vi "testionsource.vi"() -> ()   [LabVIEW 2014, in "Panels.lvlib"]
uses:
  Panels.lvlib
  CSlibraries-extern/DimLVEvent/DimIndicators/DimIndicators.lvlib
  CS_Core/CSSystem/CoreLib/CoreLib.lvlib
  CSlibraries/UtilityLib/UtilityLib.valueStatus.ctl
  CSlibraries/UtilityLib/UtilityLib.lvlib
  CSlibraries-extern/DimLVEvent/LVDimInterface/LVDimInterface.lvlib
  Instance           1 21Saved   testionsource .vi
  CSlibraries-extern/DimLVEvent/DimIndicators/DimIndicators.numericType.ctl
  CSlibraries-extern/DimLVEvent/DimIndicators/DimIndicators.numericArrayType.ctl
  CSlibraries-extern/DimLVEvent/DimIndicators/DimIndicators.anyType.ctl
panel:
  in  "SetFileLocation_Data":T1={"data"="NOLINK", "no link"=TRUE, "quality"=-1, "timeStamp"=0.0}
  in  "ISMFfreq":bool
  out "ISMFfreq_Mon":dbl=inf format="%.4f"
  in  "ISMFOffset":bool
  out "ISMFOffset_Mon":dbl=inf format="%.4f"
  in  "ISMFfreq_MonData":T2={"data"=inf, "no link"=FALSE, "quality"=1, "timeStamp"=3269018078.71}
  in  "ISMFalpha_SetValueInfoData":T3={"data"=[-1000.0, 1000.0, -1.0], "no link"=FALSE, "quality"=0, "timeStamp"=3269018078.694}
  in  "ISMFalpha_SetData":T3={"data"=[0.0, 0.0, 0.0, 0.0], "no link"=FALSE, "quality"=1, "timeStamp"=3269018077.397}
  in  "ISMFalpha_MonData":T2={"data"=inf, "no link"=TRUE, "quality"=-1, "timeStamp"=0.0}
  in  "ISMFalpha":bool
  out "ISMFalpha_Mon":dbl=inf format="%.4f"
  in  "SetFileLocation":path=path "\\\\intranet\\Files/projects/lebit/Data Exchange/data/TSTControl"
  in  "TSTBase_SetValueInfoData":T3={"data"=[-1000.0, 1000.0, -1.0], "no link"=FALSE, "quality"=0, "timeStamp"=3269018078.694}
  in  "ISMFDC":bool
  in  "ISMFamp":bool
  in  "ISMFDC_SetValueInfoData":T3={"data"=[0.0, 10.0, -1.0], "no link"=FALSE, "quality"=0, "timeStamp"=3269018078.71}
  out "i ref out":refnum<vi>
  in  "Last Loaded File_Data":T1={"data"="NOLINK", "no link"=TRUE, "quality"=-1, "timeStamp"=0.0}
  out "FileUpToDate":bool=TRUE caption="Parameter Changed"
  in  "Close All Panels":bool
  in  "ISMFfreq_SetValueInfoData":T3={"data"=[0.0, 10.0, -1.0], "no link"=FALSE, "quality"=0, "timeStamp"=3269018078.694}
  in  "ISMFOffset_SetValueInfoData":T3={"data"=[-10.0, 10.0, -1.0], "no link"=FALSE, "quality"=0, "timeStamp"=3269018078.71}
  in  "ISMFamp_SetValueInfoData":T3={"data"=[0.0, 10.0, -1.0], "no link"=FALSE, "quality"=0, "timeStamp"=3269018078.694}
  in  "ISMFamp_SetData":T3={"data"=[0.0, 0.0, 0.0, 0.0], "no link"=FALSE, "quality"=1, "timeStamp"=3269018077.507}
  in  "ISMFOffset_SetData":T3={"data"=[0.0, 0.0, 0.0, 0.0], "no link"=FALSE, "quality"=1, "timeStamp"=3269018077.507}
  in  "ISMFfreq_SetData":T3={"data"=[0.0, 0.0, 0.0, 0.0], "no link"=FALSE, "quality"=1, "timeStamp"=3269018077.507}
  in  "ISMFDC_SetData":T3={"data"=[0.0, 0.0, 0.0, 0.0], "no link"=FALSE, "quality"=1, "timeStamp"=3269018077.507}
  out "Last Loaded File":string
  in  "ISMFDC_MonData":T2={"data"=inf, "no link"=FALSE, "quality"=1, "timeStamp"=3269018078.71}
  in  "ISMFamp_MonData":T2={"data"=inf, "no link"=FALSE, "quality"=1, "timeStamp"=3269018078.694}
  in  "ISMFOffset_MonData":T2={"data"=inf, "no link"=FALSE, "quality"=1, "timeStamp"=3269018078.71}
  out "ISMFDC_Mon":dbl=inf format="%.4f"
  out "ISMFamp_Mon":dbl=inf format="%.4f"
  # "Parameter changed, data file is no longer up-to-date."
  # "Values in italic don't have a real monitor"
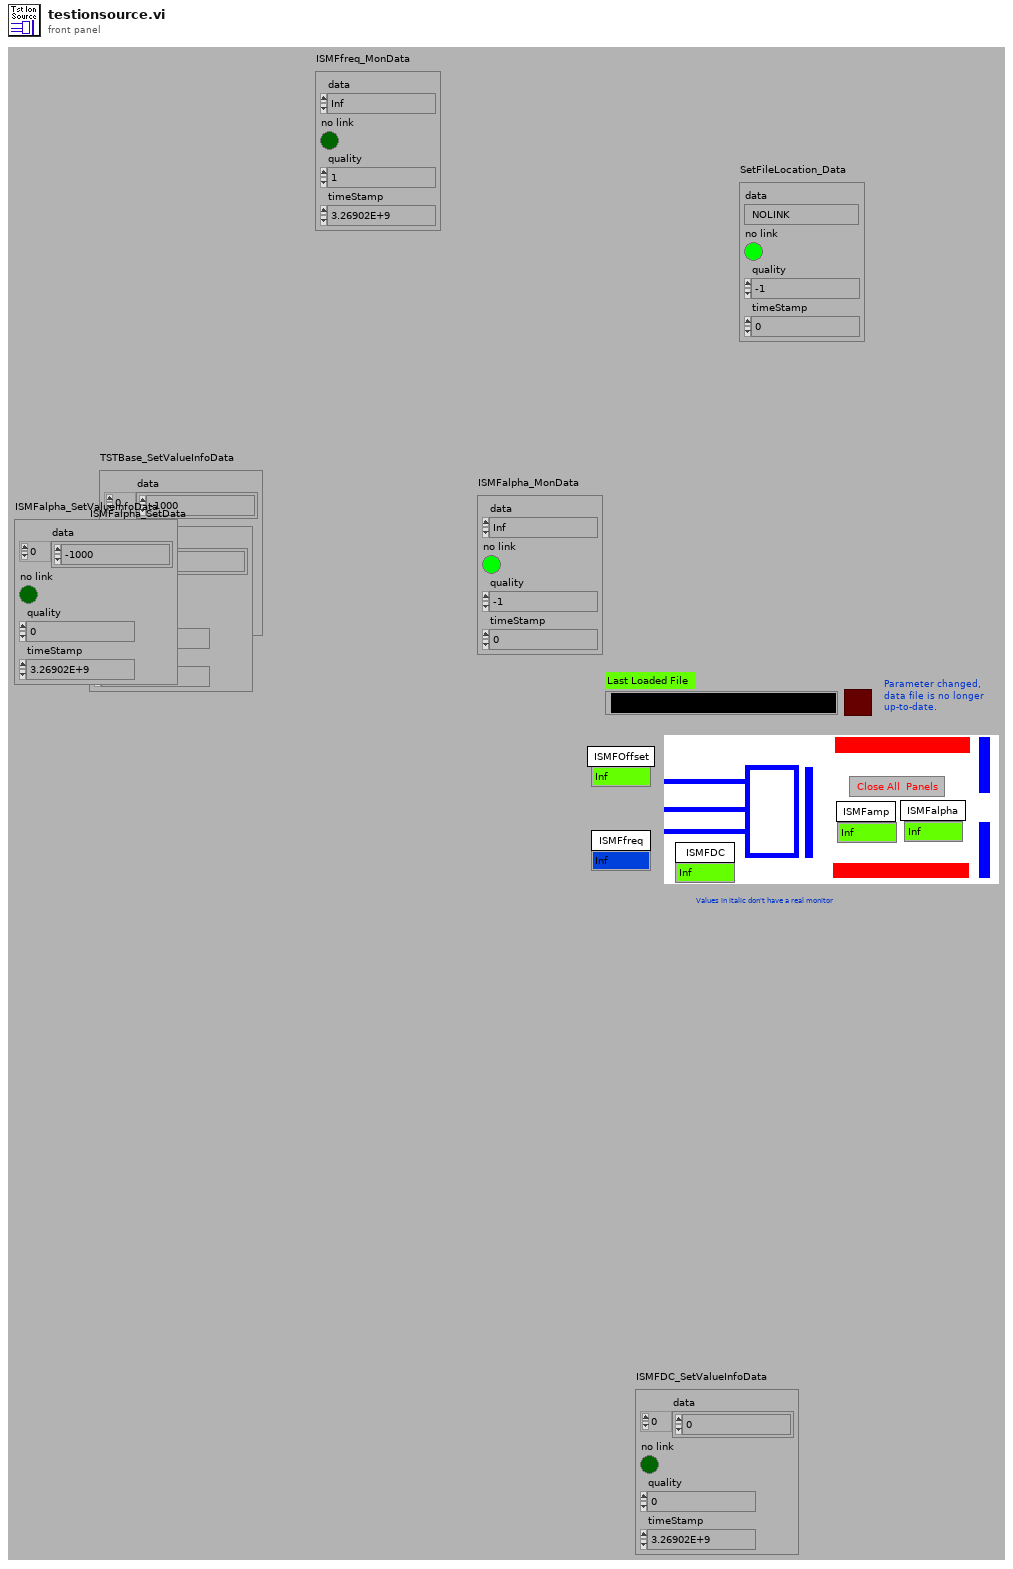
[diagram p1: front panel]
types:
  T1 = typedef "DimIndicators.lvlib/DimIndicators.anyType.ctl" = cluster{"data":string, "no link":bool, "quality":i32, "timeStamp":dbl}
  T2 = typedef "DimIndicators.lvlib/DimIndicators.numericType.ctl" = cluster{"data":dbl, "no link":bool, "quality":i32, "timeStamp":dbl}
  T3 = typedef "DimIndicators.lvlib/DimIndicators.numericArrayType.ctl" = cluster{"data":dbl[], "no link":bool, "quality":i32, "timeStamp":dbl}
  T4 = typedef "UtilityLib.lvlib/UtilityLib.valueStatus.ctl" = enum16{"no info available", "stand by/off", "on", "warning", "alarm/malfunction", "not implemented", "user action required", "important information", "system default", "control default", "indicator default", "button default"}
  T5 = cluster{"data":string, "no link":bool, "quality":i32, "timeStamp":dbl}
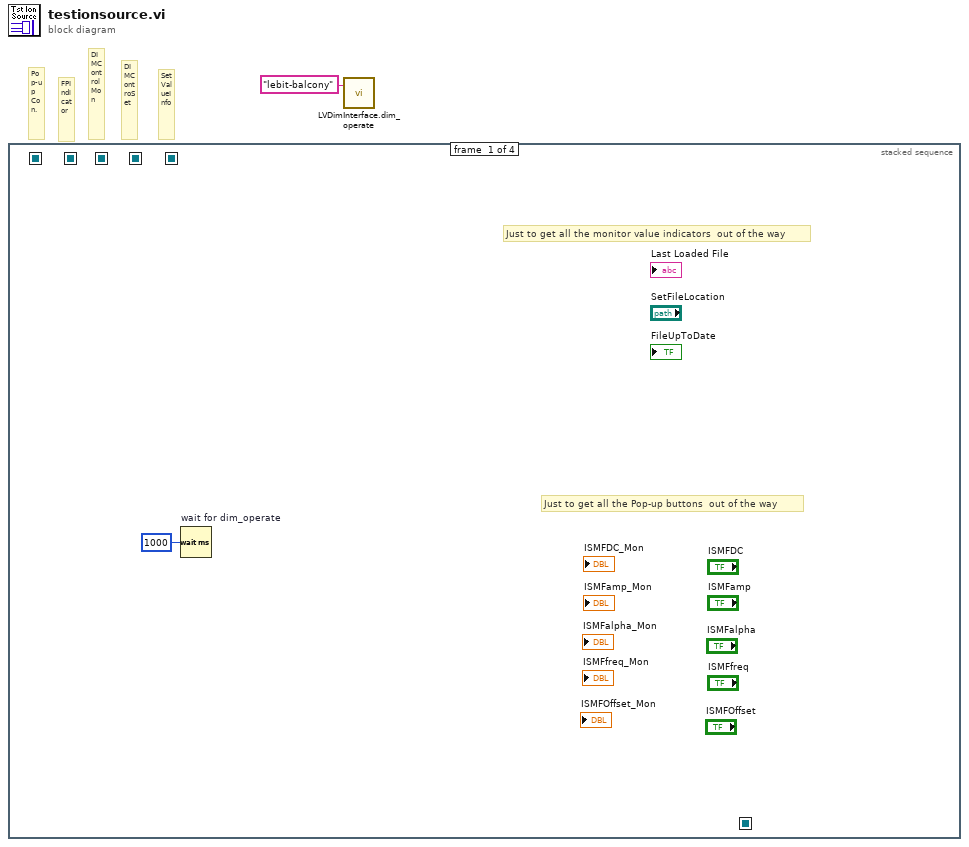
[diagram p0: block diagram]
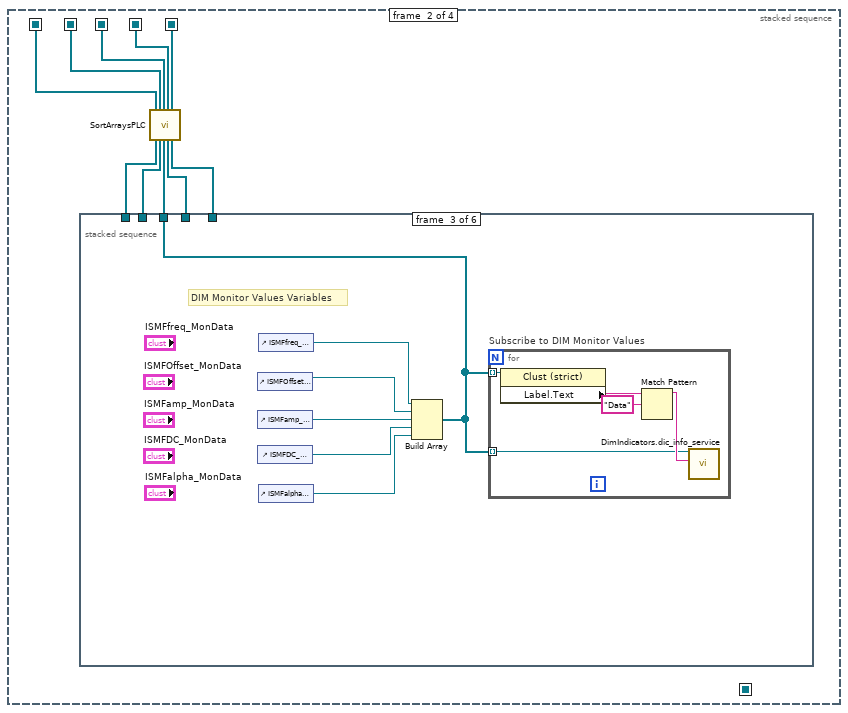
[diagram p2: hidden frame]
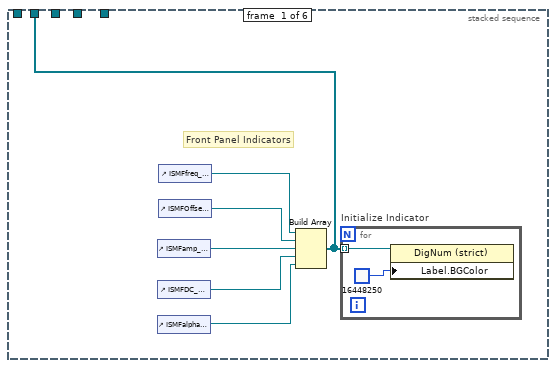
[diagram p3: hidden frame]
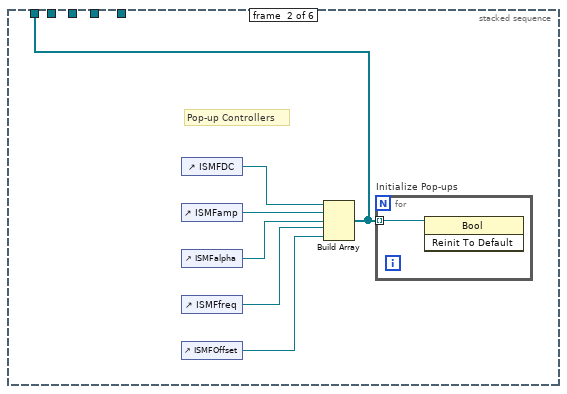
[diagram p4: hidden frame]
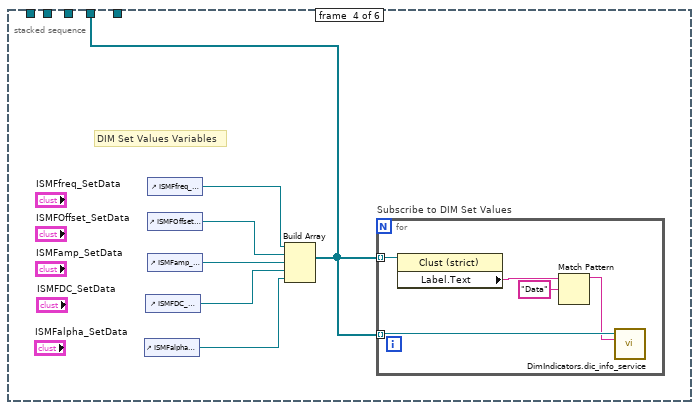
[diagram p5: hidden frame]
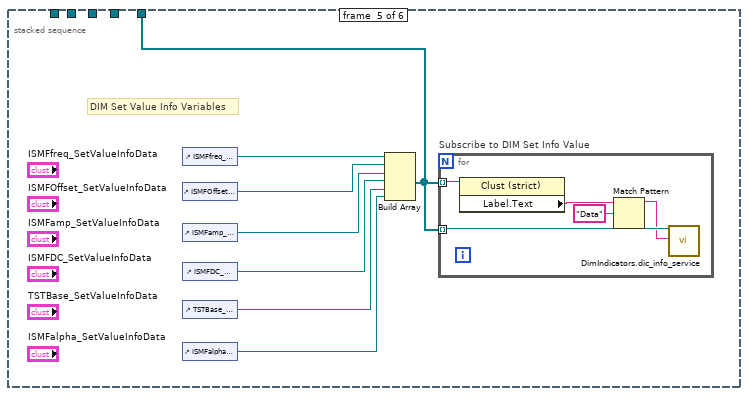
[diagram p6: hidden frame]
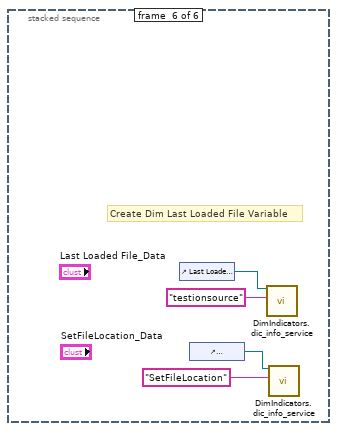
[diagram p7: hidden frame]
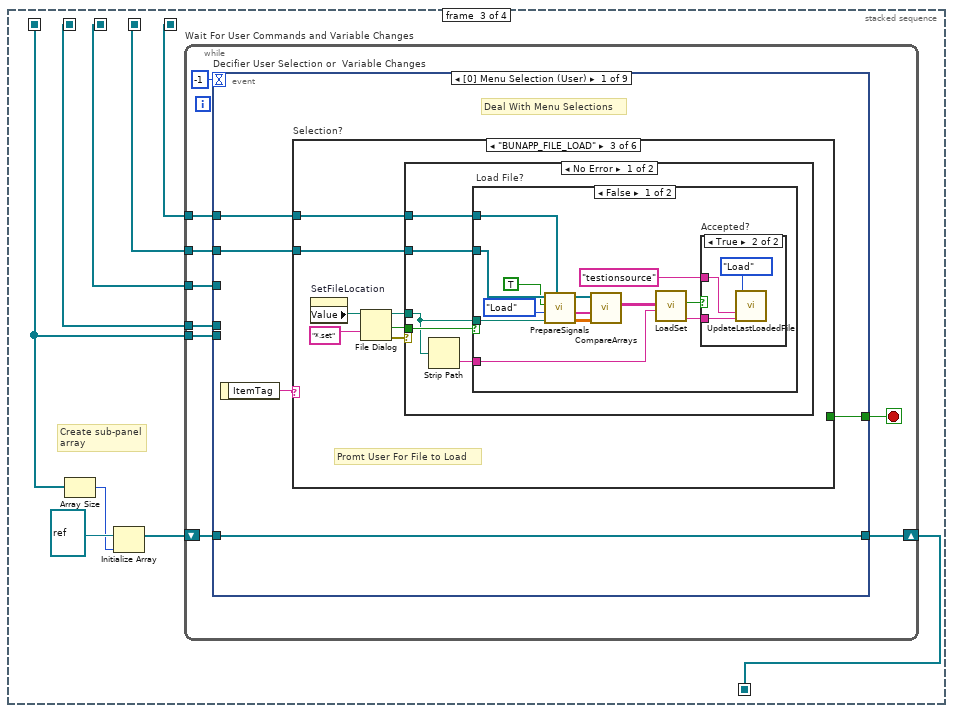
[diagram p8: hidden frame]
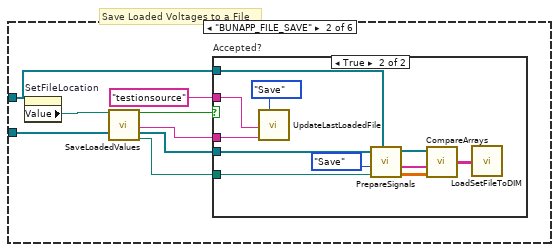
[diagram p10: hidden frame]
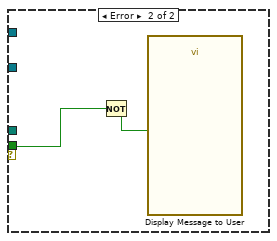
[diagram p14: hidden frame]
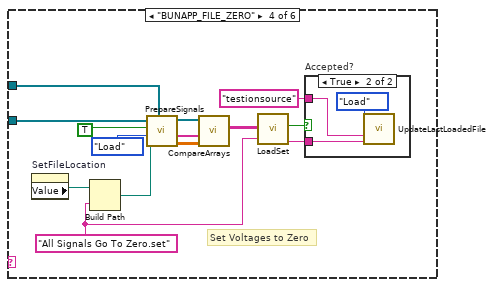
[diagram p15: hidden frame]
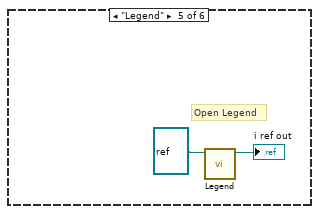
[diagram p17: hidden frame]
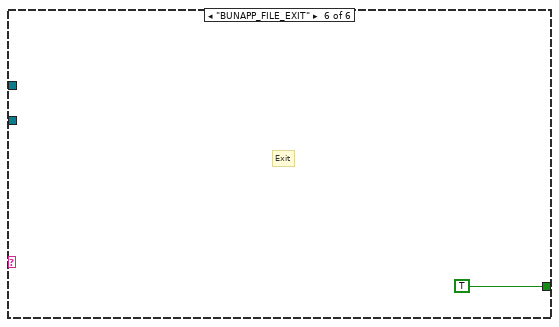
[diagram p18: hidden frame]
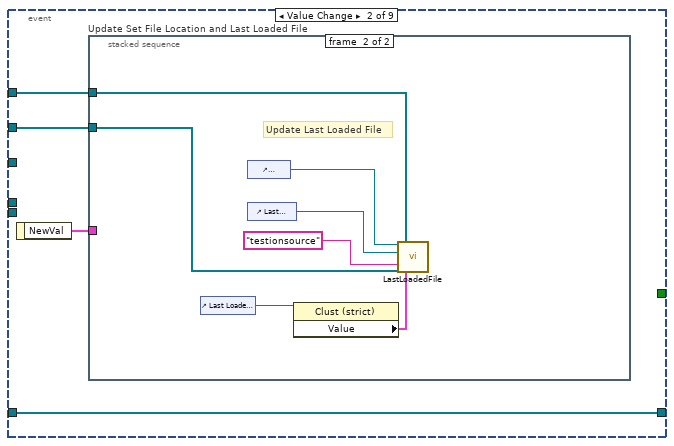
[diagram p19: hidden frame]
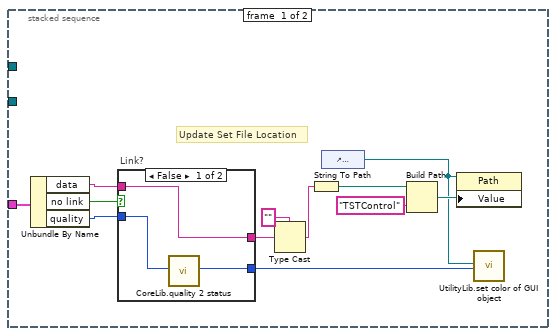
[diagram p20: hidden frame]
diagram:
  # "Pop-up Con."
  # "SetValueInfo"
  # "DIMControSet"
  # "DIMControlMon"
  # "FPIndicator"
  n1 = stacked-sequence {
    seq-local: [_ w6 _ _] -> [_ _ w71 _]
    seq-local: [_ w5 _ _] -> [_ _ w74 w268]
    seq-local: [_ _ w69 _] -> [_ _ _ w271]
    seq-local: [_ w4 _ _] -> [_ _ w68 w269]
    seq-local: [_ w3 _ _] -> [_ _ w67 w270]
    seq-local: [_ w7 _ _] -> [_ _ w66 _]
    frame #0 {
      # "Just to get all the Pop-up buttons  out of the way"
      # "Just to get all the monitor value indicators  out of the way"
      n2 = Wait (ms) "wait for dim_operate"(milliseconds to wait=u32 1000) -> ()  [unwired: 1 out]
    }
    frame #1 {
      # "Arrange references to all monitor-value related buttons into an array."
      n3 = stacked-sequence {
        tunnel: [w13 _ _ _ _ _] -> w11
        tunnel: [_ w21 _ _ _ _] -> w12
        tunnel: [_ _ w28 _ _ _] -> w10
        tunnel: [_ _ _ w39 _ _] -> w9
        tunnel: [_ _ _ _ w50 _] -> w8
        frame #0 {
          # "Front Panel Indicators"
          n4 = control-ref of="ISMFamp_Mon"() -> (w16:refnum<vi>)
          n5 = control-ref of="ISMFDC_Mon"() -> (w18:refnum<vi>)
          n6 = control-ref of="ISMFalpha_Mon"() -> (w17:refnum<vi>)
          n7 = control-ref of="ISMFfreq_Mon"() -> (w14:refnum<vi>)
          n8 = control-ref of="ISMFOffset_Mon"() -> (w15:refnum<vi>)
          n9 = Build Array(w14, w15, w16, w18, w17) -> (w13:refnum<vi>[])
          n10 = for "Initialize Indicator" {
            tunnel: w13 -> [w20] mode=indexing
            n11 = property on="Property Node" class="DigNum (strict)"(reference=w20, "Label.BGColor"=u32 16448250 ("Color Box")) -> ()  [unwired: 1 in, 2 out]
          }
        }
        frame #1 {
          # "Pop-up Controllers"
          n12 = control-ref of="ISMFDC"() -> (w26:refnum<vi>)
          n13 = control-ref of="ISMFamp"() -> (w25:refnum<vi>)
          n14 = control-ref of="ISMFalpha"() -> (w24:refnum<vi>)
          n15 = control-ref of="ISMFfreq"() -> (w23:refnum<vi>)
          n16 = control-ref of="ISMFOffset"() -> (w22:refnum<vi>)
          n17 = Build Array(w26, w25, w24, w23, w22) -> (w21:refnum<vi>[])
          n18 = for "Initialize Pop-ups" {
            tunnel: w21 -> [w27] mode=indexing
            n19 = invoke class="Bool" method="Reinit To Default"(reference=w27) -> ()  [unwired: 2 in, 3 out]
          }
        }
        frame #2 {
          # "DIM Monitor Values Variables"
          n20 = control-ref of="ISMFOffset_MonData"() -> (w33:refnum<vi>)
          n21 = control-ref of="ISMFamp_MonData"() -> (w32:refnum<vi>)
          n22 = control-ref of="ISMFDC_MonData"() -> (w31:refnum<vi>)
          n23 = control-ref of="ISMFfreq_MonData"() -> (w29:refnum<vi>)
          n24 = control-ref of="ISMFalpha_MonData"() -> (w30:refnum<vi>)
          n25 = Build Array(w29, w33, w32, w31, w30) -> (w28:refnum<vi>[])
          n26 = for "Subscribe to DIM Monitor Values" {
            tunnel: w28 -> [w35] mode=indexing
            tunnel: w28 -> [w34] mode=indexing
            n27 = property class="Clust (strict)"(reference=w34) -> ("Label.Text"=w37:string)  [unwired: 1 in, 2 out]
            n28 = Match Pattern(string=w37, regular expression="Data") -> (before substring=w36:string)  [unwired: 1 in, 3 out]
            n29 = call "DimIndicators.dic_info_service.vi"("controlRef"=w35, "serviceName"=w36) -> ()  [unwired: 16 in, 2 out]
          }
        }
        frame #3 {
          # "DIM Set Values Variables"
          n30 = control-ref of="ISMFalpha_SetData"() -> (w40:refnum<vi>)
          n31 = control-ref of="ISMFDC_SetData"() -> (w41:refnum<vi>)
          n32 = control-ref of="ISMFfreq_SetData"() -> (w44:refnum<vi>)
          n33 = control-ref of="ISMFOffset_SetData"() -> (w43:refnum<vi>)
          n34 = control-ref of="ISMFamp_SetData"() -> (w42:refnum<vi>)
          n35 = Build Array(w44, w43, w42, w41, w40) -> (w39:refnum<vi>[])
          n36 = for "Subscribe to DIM Set Values" {
            tunnel: w39 -> [w45] mode=indexing
            tunnel: w39 -> [w49] mode=indexing
            n37 = property class="Clust (strict)"(reference=w45) -> ("Label.Text"=w48:string)  [unwired: 1 in, 2 out]
            n38 = Match Pattern(string=w48, regular expression="Data") -> (before substring=w46:string)  [unwired: 1 in, 3 out]
            n39 = call "DimIndicators.dic_info_service.vi"("controlRef"=w49, "serviceName"=w46) -> ()  [unwired: 16 in, 2 out]
          }
        }
        frame #4 {
          # "DIM Set Value Info Variables"
          n40 = control-ref of="ISMFfreq_SetValueInfoData"() -> (w56:refnum<vi>)
          n41 = control-ref of="ISMFOffset_SetValueInfoData"() -> (w55:refnum<vi>)
          n42 = control-ref of="ISMFamp_SetValueInfoData"() -> (w54:refnum<vi>)
          n43 = control-ref of="ISMFDC_SetValueInfoData"() -> (w53:refnum<vi>)
          n44 = control-ref of="TSTBase_SetValueInfoData"() -> (w52:refnum<vi>)
          n45 = control-ref of="ISMFalpha_SetValueInfoData"() -> (w51:refnum<vi>)
          n46 = Build Array(w56, w55, w54, w53, w52, w51) -> (w50:refnum<vi>[])
          n47 = for "Subscribe to DIM Set Info Value" {
            tunnel: w50 -> [w57] mode=indexing
            tunnel: w50 -> [w61] mode=indexing
            n48 = property class="Clust (strict)"(reference=w57) -> ("Label.Text"=w60:string)  [unwired: 1 in, 2 out]
            n49 = Match Pattern(string=w60, regular expression="Data") -> (before substring=w58:string)  [unwired: 1 in, 3 out]
            n50 = call "DimIndicators.dic_info_service.vi"("controlRef"=w61, "serviceName"=w58) -> ()  [unwired: 16 in, 2 out]
          }
        }
        frame #5 {
          # "Create Dim Last Loaded File Variable"
          n51 = control-ref of="Last Loaded File_Data"() -> (w64:refnum<vi>)
          n52 = control-ref of="SetFileLocation_Data"() -> (w62:refnum<vi>)
          n53 = call "DimIndicators.dic_info_service.vi"("controlRef"=w64, "serviceName"="testionsource" ("string")) -> ()  [unwired: 16 in, 2 out]
          n54 = call "DimIndicators.dic_info_service.vi"("controlRef"=w62, "serviceName"="SetFileLocation" ("string")) -> ()  [unwired: 16 in, 2 out]
        }
      }
      n55 = call "SortArraysPLC.vi"("Pop-up Con."=w12, "FPIndicator in"=w11, "DIMControlMon"=w10, "DIMControSet"=w9, "SetValueInfo"=w8) -> ("Pop-up Con. out"=w7:refnum<vi>[], "FPIndicator out"=w6:refnum<vi>[], "DIMControlMon out"=w5:refnum<vi>[], "DIMControSet out"=w4:refnum<vi>[], "SetValueInfo out"=w3:refnum<vi>[])  [unwired: 18 in]
    }
    frame #2 {
      # "Create sub-panel\narray"
      n56 = Array Size(array=w66) -> (size(s)=w70:i32)
      n57 = Initialize Array(refnum<vi> refnum ("vi reference"), w70) -> (w73:refnum<vi>[])
      n58 = while "Wait For User Commands and Variable Changes" {
        tunnel: w74 -> [w82]
        tunnel: w71 -> [w81]
        shift-right: [w79] -> w69
        shift-left: w73 -> [w80]
        tunnel: w68 -> [w78]
        tunnel: w67 -> [w77]
        tunnel: w66 -> [w75]
        stop <- w83 stop-if-true
        n59 = event "Decifier User Selection or  Variable Changes" shown="[0] Menu Selection (User)" {
          selector: _ -> [_ _ _ _ _ _ _ _ _]
          dyn-events: _ -> [_ _ _ _ _ _ _ _ _]
          timeout: -1 -> [_ _ _ _ _ _ _ _ _]
          tunnel: [w85 _ _ _ _ _ _ _ _] -> w83
          tunnel: w82 -> [_ _ _ _ _ _ _ _ w245]
          tunnel: w81 -> [_ _ _ w195 _ _ _ _ _]
          tunnel: w80 -> [w88 w161 w192 w194 w222 w230 w237 w243 w244]
          tunnel: [w88 w161 w192 w194 w222 w228 w235 w243 _] -> w79
          tunnel: w78 -> [w86 w159 w190 _ w220 _ _ _ w246]
          tunnel: w77 -> [w84 w158 w186 _ _ _ _ _ w247]
          tunnel: w75 -> [_ _ _ _ _ w224 _ _ _]
          event Menu Selection (User) {
            # "Deal With Menu Selections"
            n60 = event-data() -> ("ItemTag"=w87:string)  [unwired: 1 in]
            n61 = case "Selection?" shown="\"BUNAPP_FILE_LOAD\"" w87 {
              tunnel: w86 -> [_ w93 w113 w151 _ _]
              tunnel: [_ _ _ _ _ TRUE ("stop")] -> w85
              tunnel: w84 -> [_ w89 w108 w138 _ _]
              frame "False", Default {
              }
              frame "BUNAPP_FILE_SAVE" {
                # "Save Loaded Voltages to a File"
                n62 = property on="SetFileLocation" class="Path"() -> ("Value"=w94:path)  [unwired: 2 in, 2 out]
                n63 = call "SaveLoadedValues.vi"("Panel Location?"=w94, "DIMControlSet in"=w93) -> ("File Saved?"=w95:bool, "File Name"=w92:string, "DIMControlSet out"=w90:refnum<vi>[], "Path"=w91:path)  [unwired: 14 in]
                n64 = case "Accepted?" shown="True" w95 {
                  tunnel: w92 -> [_ w105]
                  tunnel: "testionsource" ("string") -> [_ w107]
                  tunnel: w90 -> [_ w106]
                  tunnel: w91 -> [_ w104]
                  tunnel: w89 -> [_ w98]
                  frame False {
                  }
                  frame True {
                    n65 = call "UpdateLastLoadedFile.vi"("LoadOrSave"=enum16{"Load", "Save"}."Save", "GUIName"=w107, "FileNameIn"=w105) -> ()  [unwired: 13 in]
                    n66 = call "PrepareSignals.vi"("SetValueInfo in"=w98, "setfile path"=w104, "Enum"=enum16{"Save", "Load"}."Save", "DIMControSet in"=w106) -> ("indexed loaded Array"=w102:dbl[][], "Name Array"=w103:string[], "DIMControSet out"=w101:refnum<vi>[])  [unwired: 5 in]
                    n67 = call "CompareArrays.vi"("indexed loaded Array"=w102, "Name Array"=w103, "DIMControSet"=w101) -> ("Table for loading values"=w100:string[][])  [unwired: 4 in]
                    n68 = call "LoadSetFileToDIM.vi"("output array"=w100) -> ()  [unwired: 2 in]
                  }
                }
              }
              frame "BUNAPP_FILE_LOAD" {
                # "Promt User For File to Load"
                n69 = property on="SetFileLocation" class="Path"() -> ("Value"=w110:path)  [unwired: 2 in, 2 out]
                n70 = File Dialog(6:"*.set" ("pattern (all files)"), 11:w110) -> (0:w109:errorcluster, 1:w114:bool, 3:w111:path)  [unwired: 5 in, 1 out]
                n71 = case shown="No Error" w109 {
                  tunnel: w114 -> [w119 w136]
                  tunnel: w113 -> [w118 _]
                  tunnel: w111 -> [w116 _]
                  tunnel: w108 -> [w115 _]
                  frame No Error {
                    n72 = Strip Path(path=w116) -> (name=w117:string)  [unwired: 1 out]
                    n73 = case "Load File?" shown="False" w119 {
                      tunnel: w118 -> [w132 _]
                      tunnel: w117 -> [w126 _]
                      tunnel: w116 -> [w127 _]
                      tunnel: w115 -> [w120 _]
                      frame False {
                        n74 = call "PrepareSignals.vi"("SetValueInfo in"=w120, "setfile path"=w127, "Enum"=enum16{"Save", "Load"}."Load", "Display Message to \nUser"=TRUE ("Display Message to \nUser"), "DIMControSet in"=w132) -> ("indexed loaded Array"=w130:dbl[][], "Name Array"=w129:string[], "DIMControSet out"=w131:refnum<vi>[])  [unwired: 4 in]
                        n75 = call "CompareArrays.vi"("indexed loaded Array"=w130, "Name Array"=w129, "DIMControSet"=w131) -> ("Table for loading values"=w128:string[][])  [unwired: 4 in]
                        n76 = call "LoadSet.vi"("File Name In"=w126, "output array"=w128) -> ("File Name out"=w125:string, "Accepted"=w124:bool)  [unwired: 8 in]
                        n77 = case "Accepted?" shown="True" w124 {
                          tunnel: w125 -> [_ w135]
                          tunnel: "testionsource" ("string") -> [_ w134]
                          frame False {
                          }
                          frame True {
                            n78 = call "UpdateLastLoadedFile.vi"("LoadOrSave"=enum16{"Load", "Save"}."Load", "GUIName"=w134, "FileNameIn"=w135) -> ()  [unwired: 13 in]
                          }
                        }
                      }
                      frame True {
                      }
                    }
                  }
                  frame Error {
                    n79 = Not(x=w136) -> (.not. x?=w137:bool)
                    n80 = call "Display Message to User"("Enable"=w137) -> ()  [unwired: 9 in, 2 out]
                  }
                }
              }
              frame "BUNAPP_FILE_ZERO" {
                w142 = "All Signals Go To Zero.set" ("File Name")
                # "Set Voltages to Zero"
                n81 = property on="SetFileLocation" class="Path"() -> ("Value"=w140:path)  [unwired: 2 in, 2 out]
                n82 = Build Path(base path=w140, name or relative path=w142) -> (appended path=w141:path)
                n83 = call "PrepareSignals.vi"("SetValueInfo in"=w138, "setfile path"=w141, "Enum"=enum16{"Save", "Load"}."Load", "Display Message to \nUser"=TRUE ("Display Message to \nUser"), "DIMControSet in"=w151) -> ("indexed loaded Array"=w149:dbl[][], "Name Array"=w148:string[], "DIMControSet out"=w150:refnum<vi>[])  [unwired: 4 in]
                n84 = call "CompareArrays.vi"("indexed loaded Array"=w149, "Name Array"=w148, "DIMControSet"=w150) -> ("Table for loading values"=w147:string[][])  [unwired: 4 in]
                n85 = call "LoadSet.vi"("File Name In"=w142, "output array"=w147) -> ("File Name out"=w145:string, "Accepted"=w146:bool)  [unwired: 8 in]
                n86 = case "Accepted?" shown="True" w146 {
                  tunnel: w145 -> [_ w154]
                  tunnel: "testionsource" ("string") -> [_ w153]
                  frame False {
                  }
                  frame True {
                    n87 = call "UpdateLastLoadedFile.vi"("LoadOrSave"=enum16{"Load", "Save"}."Load", "GUIName"=w153, "FileNameIn"=w154) -> ()  [unwired: 13 in]
                  }
                }
              }
              frame "Legend" {
                # "Open Legend"
                n88 = call "Legend.vi"("i ref in"=refnum<vi> refnum) -> ("i ref out"=→"i ref out":refnum<vi>)  [unwired: 10 in]
              }
              frame "BUNAPP_FILE_EXIT" {
                # "Exit"
              }
            }
          }
          event Value Change {
            n89 = event-data() -> ("NewVal"=w160:T1)  [unwired: 1 in]
            n90 = stacked-sequence "Update Set File Location and Last Loaded File" {
              tunnel: w160 -> [w163 _]
              tunnel: w159 -> [_ w181]
              tunnel: w158 -> [_ w179]
              frame #0 {
                # "Update Set File Location"
                n91 = Unbundle By Name(w163) -> ("data"=w172:string, "no link"=w171:bool, "quality"=w170:i32)
                n92 = case "Link?" shown="False" w171 {
                  tunnel: w170 -> [w176 _]
                  tunnel: [w175 UtilityLib.valueStatus."no info available" ("valueStatus")] -> w173
                  tunnel: w172 -> [w174 _]
                  tunnel: [w174 w177] -> w168
                  frame False {
                    n93 = call "CoreLib.quality 2 status.vi"("quality"=w176) -> ("valueStatus"=w175:T4)  [unwired: 18 in]
                  }
                  frame True {
                    n94 = call "EmptyString.vi"() -> ("String"=w177:string)
                  }
                }
                n95 = Type Cast(type="" ("regular expression"), x=w168) -> (*(type *) &x=w167:string)
                n96 = String To Path(string=w167) -> (path=w164:path)
                n97 = control-ref of="SetFileLocation"() -> (w162:refnum<vi>)
                n98 = Build Path(base path=w164, name or relative path="TSTControl") -> (appended path=w165:path)
                n99 = property class="Path"(reference=w162, "Value"=w165) -> ()  [unwired: 1 in, 2 out]
                n100 = call "UtilityLib.set color of GUI object.vi"("GUI object Ref"=w162, "valueStatus"=w173) -> ()  [unwired: 17 in, 1 out]
              }
              frame #1 {
                # "Update Last Loaded File"
                n101 = control-ref of="Last Loaded File_Data"() -> (w180:refnum<vi>)
                n102 = control-ref of="SetFileLocation"() -> (w183:refnum<vi>)
                n103 = control-ref of="Last Loaded File"() -> (w182:refnum<vi>)
                n104 = property class="Clust (strict)"(reference=w180) -> ("Value"=w185:T5)  [unwired: 1 in, 2 out]
                n105 = call "LastLoadedFile.vi"("SetFileLocation"=w183, "Last Loaded File"=w182, "GUIName"="testionsource" ("string"), "DIMControSet in"=w181, "SetValueInfo in"=w179, "NewVal"=w185) -> ()  [unwired: 14 in]
              }
            }
          }
          event Value Change {
            # "Update Last Loaded File"
            n106 = event-data() -> ("NewVal"=w191:T1)  [unwired: 1 in]
            n107 = control-ref of="SetFileLocation"() -> (w189:refnum<vi>)
            n108 = control-ref of="Last Loaded File"() -> (w188:refnum<vi>)
            n109 = call "LastLoadedFile.vi"("SetFileLocation"=w189, "Last Loaded File"=w188, "GUIName"="testionsource" ("string"), "DIMControSet in"=w190, "SetValueInfo in"=w186, "NewVal"=w191) -> ()  [unwired: 14 in]
          }
          event Value Change {
            n110 = event-data() -> ("CtlRef"=w193:refnum<vi>, "NewVal"=w196:T2)  [unwired: 1 in, 4 out]
            n111 = for "Check if Indicator Exists for the Monitor Value?" {
              tunnel: w196 -> [w205]
              tunnel: w195 -> [w202] mode=indexing
              tunnel: w193 -> [w201]
              # "Updating a Monitor Value"
              n112 = property class="DigNum (strict)"(reference=w202) -> (reference out=w197:refnum<vi>, "Label.Text"=w199:string)  [unwired: 1 in, 1 out]
              n113 = property class="Clust (strict)"(reference=w201) -> ("Label.Text"=w203:string)  [unwired: 1 in, 2 out]
              n114 = Match Pattern(string=w203, regular expression="Data") -> (before substring=w198:string)  [unwired: 1 in, 3 out]
              n115 = Equal?(x=w199, y=w198) -> (x = y?=w200:bool)
              n116 = case "Indicator exists?" shown="True" w200 {
                tunnel: w205 -> [w212 _]
                tunnel: w197 -> [w206 _]
                frame True {
                  n117 = Unbundle By Name(w212) -> ("data"=w208:dbl, "no link"=w209:bool, "quality"=w211:i32)
                  n118 = case shown="False" w209 {
                    tunnel: w211 -> [w215 _]
                    tunnel: [w214 UtilityLib.valueStatus."no info available" ("valueStatus")] -> w210
                    tunnel: w208 -> [w213 _]
                    tunnel: [w213 inf] -> w207
                    frame False {
                      n119 = call "CoreLib.quality 2 status.vi"("quality"=w215) -> ("valueStatus"=w214:T4)  [unwired: 18 in]
                    }
                    frame True {
                    }
                  }
                  n120 = property class="DigNum (strict)"(reference=w206, "Value"=w207) -> ()  [unwired: 1 in, 2 out]
                  n121 = call "TextColor.vi"("valueStatus"=w210, "reference"=w206) -> ()  [unwired: 10 in]
                }
                frame False {
                }
              }
            }
          }
          event Value Change {
            n122 = event-data() -> ("CtlRef"=w221:refnum<vi>)  [unwired: 1 in, 5 out]
            n123 = property on="FileUpToDate" class="Bool (strict)"() -> ("Value"=w218:bool)  [unwired: 2 in, 2 out]
            n124 = call "FileUpToDate.vi"("FileUpToDate in"=w218, "DIMControSet out"=w220, "CtlRef"=w221) -> ("FileUpToDate out"=w219:bool)  [unwired: 16 in]
            n125 = property on="FileUpToDate" class="Bool (strict)"("Value"=w219) -> ()  [unwired: 2 in, 2 out]
          }
          event "ISMFamp", "ISMFDC", "ISMFalpha", "ISMFOffset", "ISMFfreq": Value Change {
            # "Find sub-panel index"
            # "opening or closing a sub-panel"
            n126 = event-data() -> ("CtlRef"=w223:refnum<vi>)  [unwired: 1 in, 3 out]
            n127 = Search 1D Array(1D array=w224, element=w223) -> (index of element=w229:i32)  [unwired: 1 in]
            n128 = Index Array(array=w230, index=w229) -> (element=w227:refnum<vi>)
            n129 = invoke class="Bool" method="Reinit To Default"(reference=w223) -> ()  [unwired: 2 in, 3 out]
            n130 = property class="VI"(reference=w227) -> ("Front Panel.Open"=w226:bool)  [unwired: 1 in, 2 out]
            n131 = case "Panel Already Open?" shown="False" w226 {
              tunnel: w223 -> [w231 _]
              tunnel: w227 -> [_ w234]
              tunnel: [w232 refnum<vi> refnum ("vi reference")] -> w225
              frame False {
                n132 = call "OpenPanel.vi"("CtlRef"=w231) -> ("vi reference"=w232:refnum<vi>)  [unwired: 2 in]
              }
              frame True {
                n133 = call "PanelClose.vi"("vi reference"=w234) -> ()
              }
            }
            n134 = Replace Array Subset(array=w230, new element=w225, index=w229) -> (w228:refnum<vi>[])
          }
          event "Close All Panels": Value Change {
            n135 = event-data() -> ()  [unwired: 1 in, 6 out]
            n136 = case "Close Open Panels?" shown="True" "Close All Panels" {
              tunnel: w237 -> [w238 w240]
              tunnel: [w238 w239] -> w235
              frame False {
              }
              frame True {
                n137 = for "Close Open Panels" {
                  tunnel: w240 -> [w242] mode=indexing
                  tunnel: w240 -> [w241]
                  tunnel: [w241] -> w239
                  n138 = call "PanelClose.vi"("vi reference"=w242) -> ()
                }
              }
            }
          }
          event Timeout {
            # "Timeout"
            n139 = event-data() -> ()  [unwired: 1 in, 3 out]
          }
          event Panel Close {
            n140 = event-data() -> ()  [unwired: 1 in, 4 out]
            n141 = stacked-sequence {
              tunnel: w247 -> [w252 _]
              tunnel: w246 -> [w251 _]
              tunnel: w245 -> [w250 _]
              tunnel: w244 -> [w253 _]
              frame #0 {
                # "Release DIM Services"
                n142 = for "Close Open Panels" {
                  tunnel: w253 -> [w263] mode=indexing
                  n143 = call "PanelClose.vi"("vi reference"=w263) -> ()
                }
                n144 = for "For Each Service" {
                  tunnel: w252 -> [w261] mode=indexing
                  n145 = Not A Number/Path/Refnum?(number/path/refnum=w261) -> (NaN/Path/Refnum?=w260:bool)
                  n146 = case "Not a Reference?" shown="False" w260 {
                    tunnel: w261 -> [w262 _]
                    frame False {
                      n147 = call "DimIndicators.dic_release_service.vi"("controlRef"=w262) -> ()  [unwired: 18 in, 1 out]
                    }
                    frame True {
                    }
                  }
                }
                n148 = for "For Each Service" {
                  tunnel: w251 -> [w258] mode=indexing
                  n149 = Not A Number/Path/Refnum?(number/path/refnum=w258) -> (NaN/Path/Refnum?=w257:bool)
                  n150 = case "Not a Reference?" shown="False" w257 {
                    tunnel: w258 -> [w259 _]
                    frame False {
                      n151 = call "DimIndicators.dic_release_service.vi"("controlRef"=w259) -> ()  [unwired: 18 in, 1 out]
                    }
                    frame True {
                    }
                  }
                }
                n152 = for "For Each Service" {
                  tunnel: w250 -> [w255] mode=indexing
                  n153 = Not A Number/Path/Refnum?(number/path/refnum=w255) -> (NaN/Path/Refnum?=w254:bool)
                  n154 = case "Not a Reference?" shown="False" w254 {
                    tunnel: w255 -> [w256 _]
                    frame False {
                      n155 = call "DimIndicators.dic_release_service.vi"("controlRef"=w256) -> ()  [unwired: 18 in, 1 out]
                    }
                    frame True {
                    }
                  }
                }
                n156 = control-ref of="SetFileLocation_Data"() -> (w248:refnum<vi>)
                n157 = control-ref of="Last Loaded File_Data"() -> (w249:refnum<vi>)
                n158 = call "DimIndicators.dic_release_service.vi"("controlRef"=w249) -> ()  [unwired: 18 in, 1 out]
                n159 = call "DimIndicators.dic_release_service.vi"("controlRef"=w248) -> ()  [unwired: 18 in, 1 out]
              }
              frame #1 {
                # "Close Front Panel"
                n160 = Current VI's Path() -> (path=w264:path)
                n161 = Open VI Reference(vi path=w264) -> (vi reference=w266:refnum<vi>, error out=w267:errorcluster)  [unwired: 5 in]
                n162 = property class="VI"(reference=w266, error in=w267, "Front Panel Window:Open"=FALSE) -> ()  [unwired: 2 out]
              }
            }
          }
        }
      }
    }
    frame #3 {
      n163 = stacked-sequence {
        tunnel: w271 -> [w277 _ _]
        tunnel: w269 -> [w275 _ _]
        tunnel: w270 -> [w276 _ _]
        tunnel: w268 -> [w274 _ _]
        frame #0 {
          # "Release DIM Services"
          n164 = control-ref of="Last Loaded File_Data"() -> (w273:refnum<vi>)
          n165 = control-ref of="SetFileLocation_Data"() -> (w272:refnum<vi>)
          n166 = call "DimIndicators.dic_release_service.vi"("controlRef"=w273) -> ()  [unwired: 18 in, 1 out]
          n167 = call "DimIndicators.dic_release_service.vi"("controlRef"=w272) -> ()  [unwired: 18 in, 1 out]
          n168 = for "For Each Service" {
            tunnel: w276 -> [w285] mode=indexing
            n169 = Not A Number/Path/Refnum?(number/path/refnum=w285) -> (NaN/Path/Refnum?=w284:bool)
            n170 = case "Not a Reference?" shown="False" w284 {
              tunnel: w285 -> [w286 _]
              frame False {
                n171 = call "DimIndicators.dic_release_service.vi"("controlRef"=w286) -> ()  [unwired: 18 in, 1 out]
              }
              frame True {
              }
            }
          }
          n172 = for "For Each Service" {
            tunnel: w275 -> [w282] mode=indexing
            n173 = Not A Number/Path/Refnum?(number/path/refnum=w282) -> (NaN/Path/Refnum?=w281:bool)
            n174 = case "Not a Reference?" shown="False" w281 {
              tunnel: w282 -> [w283 _]
              frame False {
                n175 = call "DimIndicators.dic_release_service.vi"("controlRef"=w283) -> ()  [unwired: 18 in, 1 out]
              }
              frame True {
              }
            }
          }
          n176 = for "For Each Service" {
            tunnel: w274 -> [w279] mode=indexing
            n177 = Not A Number/Path/Refnum?(number/path/refnum=w279) -> (NaN/Path/Refnum?=w278:bool)
            n178 = case "Not a Reference?" shown="False" w278 {
              tunnel: w279 -> [w280 _]
              frame False {
                n179 = call "DimIndicators.dic_release_service.vi"("controlRef"=w280) -> ()  [unwired: 18 in, 1 out]
              }
              frame True {
              }
            }
          }
          n180 = for "Close Open Panels" {
            tunnel: w277 -> [w287] mode=indexing
            n181 = call "PanelClose.vi"("vi reference"=w287) -> ()
          }
        }
        frame #1 {
          # "Close Front Panel"
          n182 = Current VI's Path() -> (path=w291:path)
          n183 = Open VI Reference(vi path=w291) -> (vi reference=w289:refnum<vi>, error out=w288:errorcluster)  [unwired: 5 in]
          n184 = property class="VI"(reference=w289, error in=w288, "Front Panel Window:Open"=FALSE) -> ()  [unwired: 2 out]
        }
        frame #2 {
          # "Stop Panel"
          n185 = Stop(stop? (T)=TRUE) -> ()
        }
      }
    }
  }
  n186 = call "LVDimInterface.dim_operate.vi"("DNSNode"="lebit-balcony" ("DNS node")) -> ()  [unwired: 19 in]
